vi "Complete Elliptic Integral K.vi"(11 "k":dbl format="%.2f") -> (3 "K(k)":dbl format="%.2f")   [LabVIEW 2017, in "NI_Gmath.lvlib"]
doc: "Computes the Legendre elliptic integral of the first kind. You must manually select the polymorphic instance you want to use."
uses:
  NI_Gmath.lvlib
  <resource>/lvanlys.dll
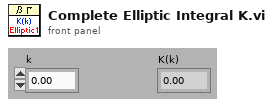
[diagram p1: front panel]
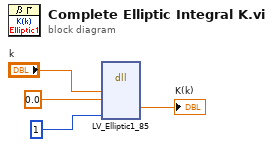
[diagram p0: block diagram]
diagram:
  n1 = dll-call lib="C:/Program Files (x86)/National Instruments/LabVIEW 2017/resource/lvanlys.*" fn="LV_Elliptic1_85"("k"="k", "a"=0.0, "funcType"=1) -> ("Elliptic1(k, a)"=→"K(k)":dbl)  [unwired: 8 in, 2 out]
